vi "FRIC_navX_Internal_Serial_ProcessingLoop.vi"(7 "Device Number":T3, 11 "Rate (4Hz-200Hz)":u8=50 min=4 max=200) -> ()   [LabVIEW 2025]
doc: "This navX VI handles the reading/writing for the navX. All of the good stuff is in here.\nTHIS VI SHOULD NOT BE CALLED BY THE USER!"
uses:
  _TypeDefs/Z900_navX_SerialStreamTypeDef.ctl
  _TypeDefs/FRIC_navX_DeviceNumbersTypeDef.ctl
  <vilib>/Rock Robotics/WPI/SerialPort/WPI_SerialPort.ctl
  _TypeDefs/Z900_navX_ProtocolTypeDef.ctl
  _TypeDefs/FRIC_navX_ProcessingLoopStatesTypeDef_I2C.ctl
  _TypeDefs/FRIC_navX_I2C Process Loop TypeDef.ctl
  _TypeDefs/Z900_navX_DeviceTypeDef.ctl
  _TypeDefs/Z900_navX_NotifyPacketTypeDef.ctl
  _TypeDefs/Z900_navX_ActionTypeDef.ctl
  <vilib>/Rock Robotics/SystemInterfaces/i2clib/i2c_bus.ctl
  _TypeDefs/Z900_navX_IntegrationControlRegisters.ctl
  <vilib>/Rock Robotics/WPI/SPI/WPI_SPIDevRef.ctl
  <vilib>/Rock Robotics/SystemInterfaces/spilib/spi_bus.ctl
  <vilib>/Rock Robotics/WPI/SerialPort/WPI_SerialPortRef.ctl
  <vilib>/Platform/TimedLoop/XDataNode/timing_clust.ctl
  <vilib>/Platform/TimedLoop/XDataNode/nitl_modes.ctl
  <vilib>/Platform/TimedLoop/XDataNode/wakeup.ctl
  <vilib>/Rock Robotics/SystemInterfaces/NetworkCommunication/NetComm_UsageReport_ResourceType.ctl
  <vilib>/Rock Robotics/SystemInterfaces/Utilities/FPGA_UtilitiesRead LocalTime.vi
  <vilib>/Platform/TimedLoop/XDataNode/XDataNode.xnode
  <vilib>/Platform/TimedLoop/XDataNode/XDNodeRunTimeDep.lvlib
panel:
  in  "Tab Control":enum32{"Page 1", "Page 2"}(tab)
  in  "Halt":bool
  out "Connected":bool
  out "error":errorcluster
  in  "Stream Type":T1=enum."AHRSAndPositioning"
  in  "Serial Port":T2=enum."MXP TTL"
  out "Loop Time":i64
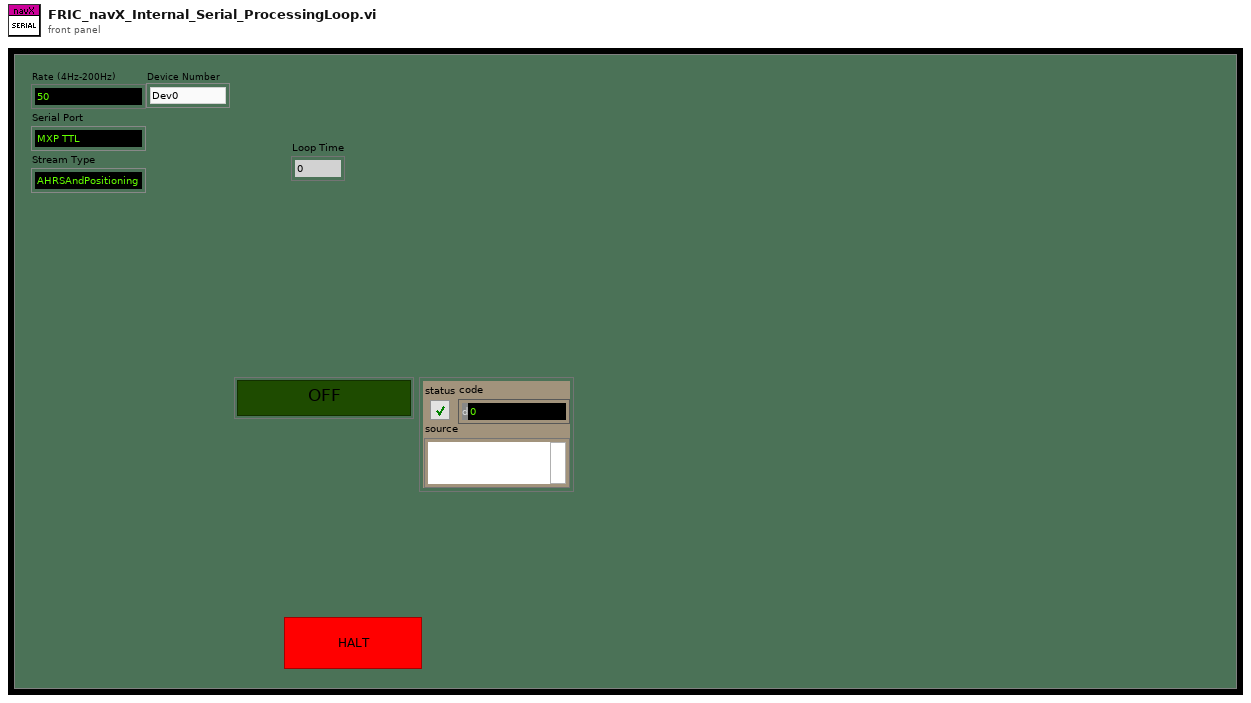
[diagram p1: front panel]
types:
  T1 = typedef "Z900_navX_SerialStreamTypeDef.ctl" = enum16{"YRPH", "Quaterinons", "Gyro/Raw", "AHRS", "AHRSAndPositioning", "AHRSAndPOSTime"}
  T2 = typedef "WPI_SerialPort.ctl" = enum16{"Onboard RS-232", "MXP TTL", "USB 1", "USB 2"}
  T3 = typedef "FRIC_navX_DeviceNumbersTypeDef.ctl" = enum16{"Dev0", "Dev1", "Dev2", "Dev3"}
  T4 = typedef "FRIC_navX_I2C Process Loop TypeDef.ctl" = cluster{"State Array":T5[], "error":errorcluster, "FPGA Cluster":cluster{"Last Valid FPGA Time":dbl, "Error Count":i32, "Initialized":bool}, "Device Info":T6, "I2CDevRef":cluster{"DevStatus":errorcluster, "Device Address":u8, "Handle":i32, "I2C Bus":T8}, "Registry":u8[], "Command Array":T9[], "Connected?":bool, "navX Device Memory Size":i32, "notification":T10, "Memory Size Set":bool, "SPIDevRef":T12, "navX Serial Open":cluster{"Stream Type":T1, "Serial Port":T2}, "SerialPortRef":T14, "Serial Read Buffer":string, "Serial Write Buffer":string[], "Device Number":T3, "navX SPI Open":cluster{"SPI Bus":T13, "Clock Rate (Hz)":dbl}, "Loop dt":i64, "current time":timestamp, "Loop Time":i64}
  T5 = typedef "FRIC_navX_ProcessingLoopStatesTypeDef_I2C.ctl" = enum16{"Process", "INI", "Check Packets Valid", "Close", "Clear VISA", "Generate Command", "Last Packet Valid", "Open", "Read", "Reset Serial", "Set Termination Char", "Update AE", "Wait", "Write", "Exit"}
  T6 = typedef "Z900_navX_DeviceTypeDef.ctl" = cluster{"Interface":cluster{"Protocol":T7, "Update Rate (4Hz-200Hz)":u8, "navX Open TypeDef":variant}, "Notify Packet":refnum<notifier>, "Loop VI Refnum":refnum<vi>, "Ready to Close Occurrence Refnum":refnum<k4>, "Name":string}
  T7 = typedef "Z900_navX_ProtocolTypeDef.ctl" = enum16{"SERIAL", "I2C", "SPI"}
  T8 = typedef "i2c_bus.ctl" = enum16{"I2C On-Board", "I2C MXP", "Invalid"}
  T9 = typedef "Z900_navX_IntegrationControlRegisters.ctl" = u8
  T10 = typedef "Z900_navX_NotifyPacketTypeDef.ctl" = cluster{"navX Action":T11, "Data":variant, "Stream Type":T1, "Device Number":T3}
  T11 = typedef "Z900_navX_ActionTypeDef.ctl" = enum16{"None", "Halt", "Normal Read", "Update Serial Protocol", "Update Rate Htz", "Zero-Yaw", "Zero-Displacement", "Zero-Velocity"}
  T12 = typedef "WPI_SPIDevRef.ctl" = cluster{"DevStatus":errorcluster, "Handle":i32, "SPI Bus":T13}
  T13 = typedef "spi_bus.ctl" = enum16{"SPI On-Board, CS0", "SPI On-Board, CS1", "SPI On-Board, CS2", "SPI On-Board, CS3", "SPI MXP", "Invalid"}
  T14 = typedef "WPI_SerialPortRef.ctl" = cluster{"DevStatus":errorcluster, "Serial Port Name":refnum<visa-resource-name>}
  T15 = typedef "XDNodeRunTimeDep.lvlib/timing_clust.ctl" = cluster{"Expected End [f-1]":u64, "Actual End [f-1]":u64, "Finished Late? [f-1]":bool, "Expected End [i-1]":u64, "Actual End [i-1]":u64, "Finished Late? [i-1]":bool, "Expected Start [i]":u64, "Actual Start [i]":u64, "Expected Start [f]":u64, "Actual Start [f]":u64, "Source Name":string, "Structure Name":string, "Period":i64, "Deadline":i64, "Offset":i64, "Start":i64, "Priority":i32, "Timeout":i32, "Mode":T16, "Wakeup Reason":T17, "Error":errorcluster, "Source Type":string, "Secondary Source Type":string, "Global End Time":u64, "Global Start Time":u64, "Frame Duration":u64, "Iteration Duration":u64, "Assigned CPU":i32, "I/O Scan Engine Mode":u32}
  T16 = typedef "XDNodeRunTimeDep.lvlib/nitl_modes.ctl" = enum32{"No Change", "Process missed periods, maintain original phase", "Discard missed periods, maintain original phase", "Process missed periods, ignore original phase", "Discard missed periods, ignore original phase"}
  T17 = typedef "XDNodeRunTimeDep.lvlib/wakeup.ctl" = enum32{"Normal", "Aborted", "Asynchronous wakeup", "Timing source error", "Timed loop error", "Timeout"}
  T18 = typedef "NetComm_UsageReport_ResourceType.ctl" = enum8{"Controller", "Module", "Language", "CANPlugin", "Accelerometer", "ADXL345", "AnalogChannel", "AnalogTrigger", "AnalogTriggerOutput", "CANJaguar", "Compressor", "Counter", "Dashboard", "DigitalInput", "DigitalOutput", "DriverStationCIO", "DriverStationEIO", "DriverStationLCD", "Encoder", "GearTooth", "Gyro", "I2C", "Framework", "Jaguar", "Joystick", "Kinect", "KinectStick", "PIDController", "Preferences", "PWM", "Relay", "RobotDrive", "SerialPort", "Servo", "Solenoid", "SPI", "Task", "Ultrasonic", "Victor", "Button", "Command", "AxisCamera", "PCVideoServer", "SmartDashboard", "Talon", "HiTechnicColorSensor", "HiTechnicAccel", "HiTechnicCompass", "SRF08", "AnalogOutput", "Victor SP", "Talon SRX", "CAN Talon SRX", "ADXL362 Accel", "ADXRS450 Gyro", "Rev SPARK", "Mindsensors SD540", "Digital Filter", "ADIS16448", "PDP", "PCM", "PigeonIMU", "Nidec Brushless", "CTRE CANifier", "CTRE TalonFX", "CTRE Future 1", "CTRE Future 2", "CTRE Future 3", "CTRE Future 4", "CTRE Future 5", "CTRE Future 6", "Linear Filter", "Xbox Controller", "USB Camera", "NavX", "Pixy", "Pixy2", "ScanseSweep", "Shuffleboard", "CAN", "Digilent DMC60", "PWM Victor SPX", "Rev SPARK MAX PWM", "Rev SPARK MAX CAN", "ADIS16470", "PIDController2", "ProfiledPIDController", "Kinematics", "Odometry", "Units", "Trapezoid Profile", "DutyCycle", "Addressable LEDs", "Fusion Venom", "CTRE Future 7", "CTRE Future 8", "CTRE Future 9", "CTRE Future 10", "CTRE Future 11", "CTRE Future 12", "CTRE Future 13", "CTRE Future 14", "Exponential Profile", "PS4 Controller", "Photon Camera", "Photon Pose Estimator", "Path Planner Path", "Path Planner Auto", "Path Finding Command", "Redux Future 1", "Redux Future 2", "Redux Future 3", "Redux Future 4", "Redux Future 5", "Rev SPARK Flex CAN", "Rev SPARK Flex PWM", "LEDPattern", "LinearQuadraticRegulator", "KalmanFilter", "PoseEstimator", "PoseEstimator3d", "LinearSystemLoop", "WPILib_future7", "WPILib_future8", "Rev_ServoHub", "YAMS", "LumenLabs_ConnectorX", "LumenLabs_ConnectorXLED"}
  T19 = cluster{"Last Valid FPGA Time":dbl, "Error Count":i32, "Initialized":bool}
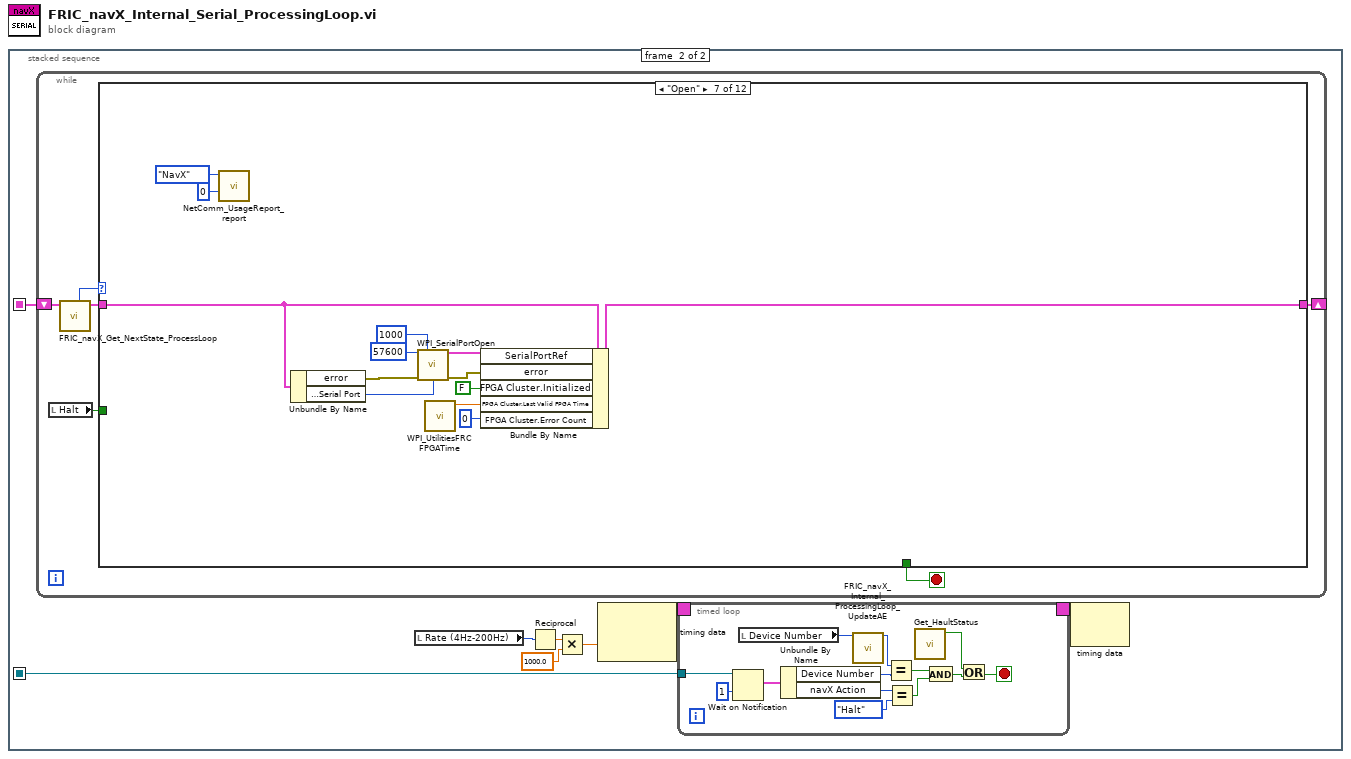
[diagram p0: block diagram]
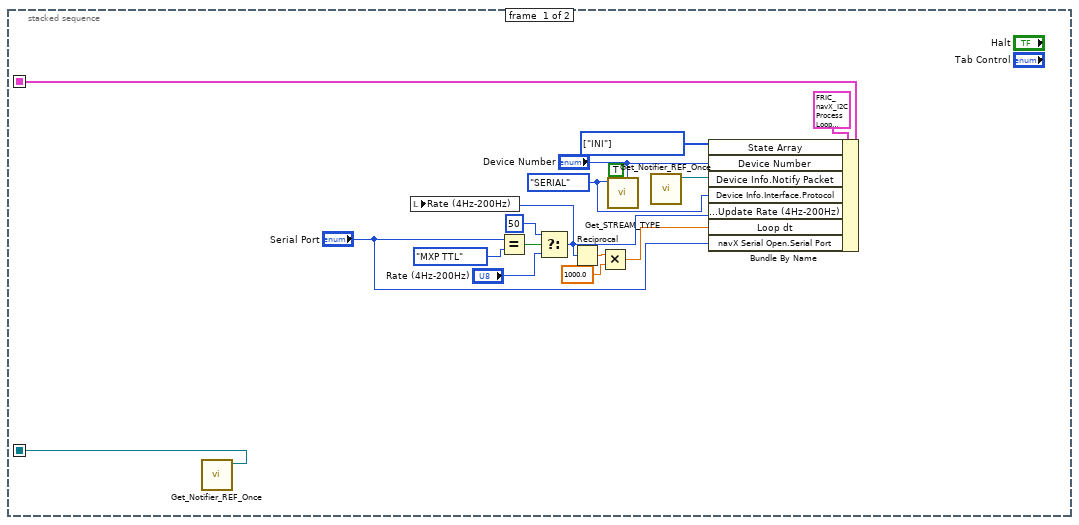
[diagram p2: hidden frame]
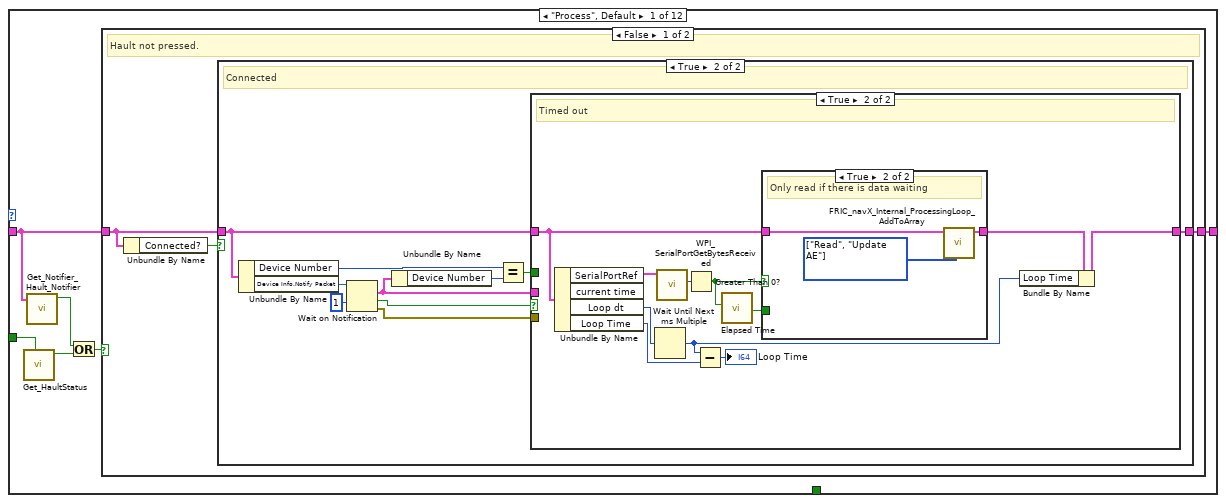
[diagram p3: hidden frame]
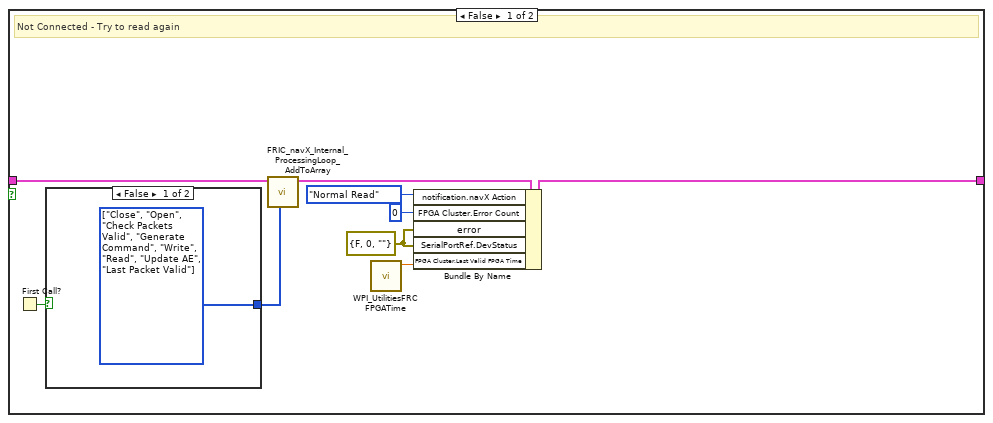
[diagram p4: hidden frame]
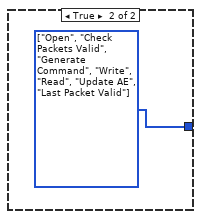
[diagram p5: hidden frame]
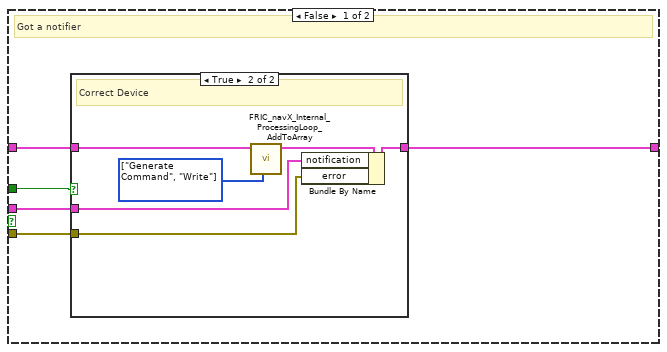
[diagram p6: hidden frame]
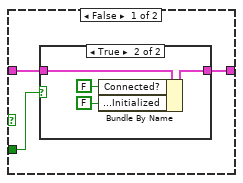
[diagram p8: hidden frame]
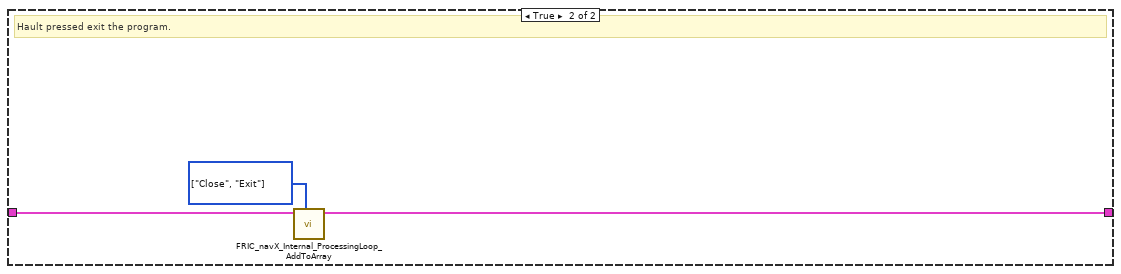
[diagram p10: hidden frame]
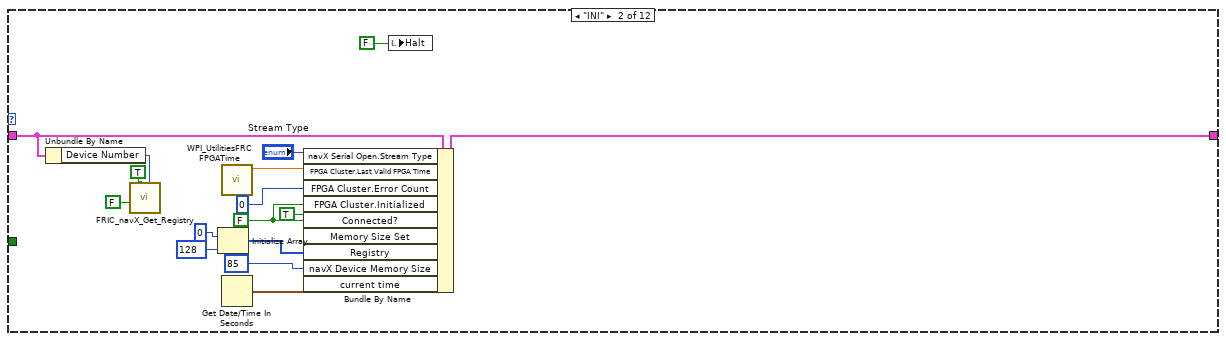
[diagram p11: hidden frame]
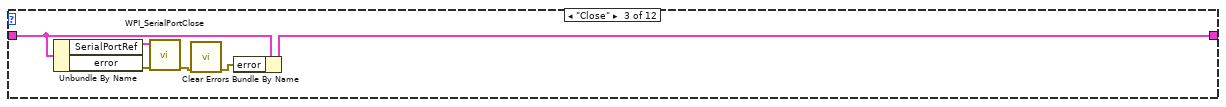
[diagram p12: hidden frame]
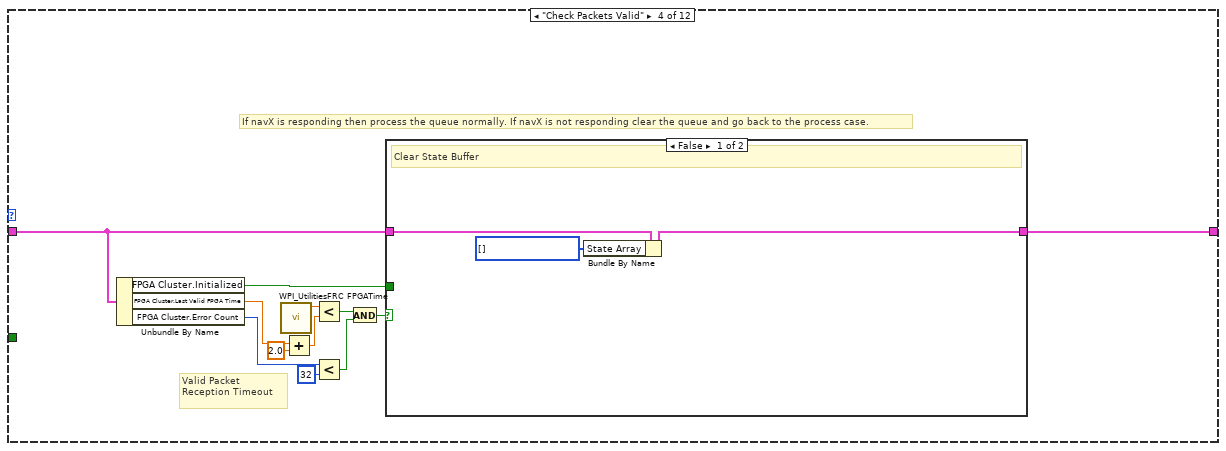
[diagram p13: hidden frame]
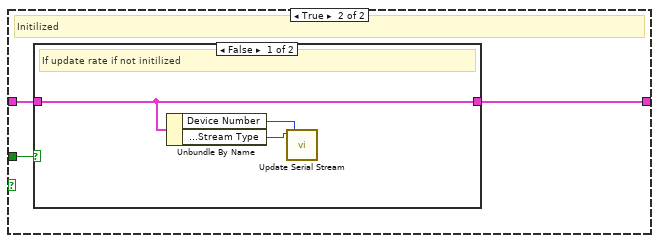
[diagram p14: hidden frame]
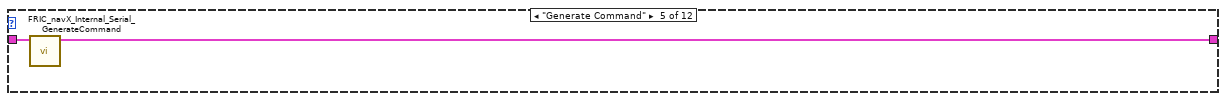
[diagram p16: hidden frame]
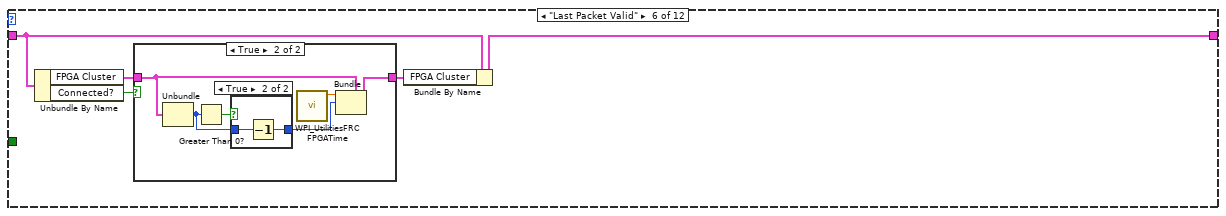
[diagram p17: hidden frame]
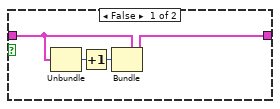
[diagram p18: hidden frame]
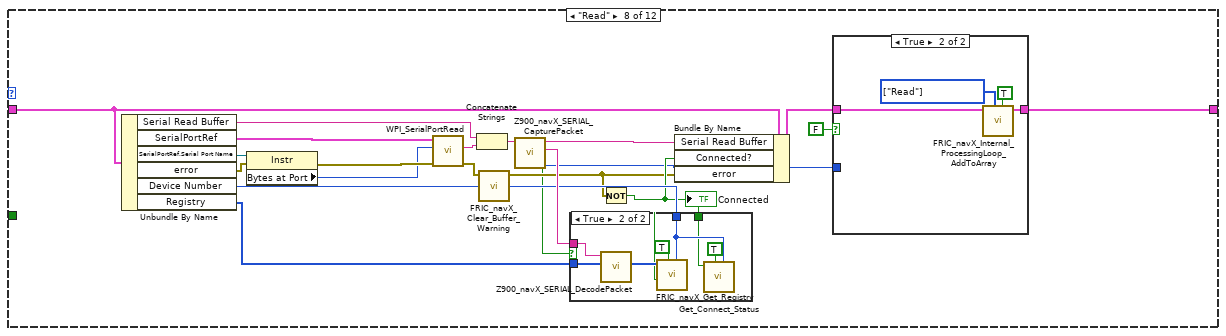
[diagram p20: hidden frame]
diagram:
  n1 = stacked-sequence {
    seq-local: [w17 _] -> [_ w25]
    seq-local: [w13 _] -> [_ w18]
    frame #0 {
      w1 = Z900_navX_ProtocolTypeDef."SERIAL" ("Protocol")
      w15 = T5[] [enum."INI"] items=["Process", "INI", "Check Packets Valid", "Close", "Clear VISA", "Generate Command", "Last Packet Valid", "Open", "Read", "Reset Serial", "Set Termination Char", "Update AE", "Wait", "Write", "Exit"] ("State Array")
      n2 = call "Get_Notifier_REF_Once.vi"() -> ("notifier ref out"=w13:refnum<notifier>)  [unwired: 10 in, 1 out]
      n3 = Equal?(x="Serial Port", y=WPI_SerialPort."MXP TTL") -> (x = y?=w11:bool)
      n4 = Select(t=u8 50, s=w11, f="Rate (4Hz-200Hz)") -> (s? t:f=w6:u8)
      n5 = local write "Rate (4Hz-200Hz)"(w6) -> ()
      n6 = Reciprocal(x=w6) -> (1/x=w9:dbl)
      n7 = Multiply(x=w9, y=1000.0) -> (x*y=w7:dbl)
      n8 = call "Get_STREAM_TYPE.vi"("Device Number"="Device Number", "Update"=TRUE, "Protocol (in)"=w1) -> ()  [unwired: 8 in, 1 out]
      n9 = call "Get_Notifier_REF_Once.vi"() -> ("notifier ref out"=w14:refnum<notifier>)  [unwired: 10 in, 1 out]
      n10 = Bundle By Name(cluster=T4 {"State Array"=[enum."INI", enum."Open"], "error"={"status"=FALSE, "code"=0, "source"=""}, "FPGA Cluster"={"Last Valid FPGA Time"=0.0, "Error Count"=0, "Initialized"=FALSE}, "Device Info"={"Interface"={"Protocol"=enum."SERIAL", "Update Rate (4Hz-200Hz)"=4, "navX Open TypeDef"=variant}, "Notify Packet"=refnum, "Loop VI Refnum"=refnum, "Ready to Close Occurrence Refnum"=refnum, "Name"=""}, "I2CDevRef"={"DevStatus"={"status"=FALSE, "code"=0, "source"=""}, "Device Address"=0, "Handle"=0, "I2C Bus"=enum."Invalid"}, "Registry"=[], "Command Array"=[214, 32], "Connected?"=FALSE, "navX Device Memory Size"=85, "notification"={"navX Action"=enum."None", "Data"=variant, "Stream Type"=enum."YRPH", "Device Number"=enum."Dev0"}, "Memory Size Set"=FALSE, "SPIDevRef"={"DevStatus"={"status"=FALSE, "code"=0, "source"=""}, "Handle"=0, "SPI Bus"=enum."SPI On-Board, CS0"}, "navX Serial Open"={"Stream Type"=enum."YRPH", "Serial Port"=enum."Onboard RS-232"}, "SerialPortRef"={"DevStatus"={"status"=FALSE, "code"=0, "source"=""}, "Serial Port Name"=""}, "Serial Read Buffer"="", "Serial Write Buffer"=[], "Device Number"=enum."Dev0", "navX SPI Open"={"SPI Bus"=enum."SPI MXP", "Clock Rate (Hz)"=500000.0}, "Loop dt"=0, "current time"=timestamp(0 s since 1904-01-01), "Loop Time"=0} ("I2C Process Loop TypeDef"), "State Array"=w15, "Device Number"="Device Number", "Device Info.Notify Packet"=w14, "Device Info.Interface.Protocol"=w1, "Device Info.Interface.Update Rate (4Hz-200Hz)"=w6, "Loop dt"=w7, "navX Serial Open.Serial Port"="Serial Port") -> (w17:T4)
    }
    frame #1 {
      n11 = while {
        shift-right: [w45] -> _
        shift-left: w25 -> [w48]
        stop <- w49 stop-if-true
        n12 = local read "Halt"() -> (w44:bool)
        n13 = call "FRIC_navX_Get_NextState_ProcessLoop.vi"("I2C Process Loop TypeDef (in)"=w48) -> ("I2C Process Loop TypeDef (out)"=w47:T4, "Current State"=w46:T5)  [unwired: 9 in]
        n14 = case shown="\"Open\"" w46 {
          tunnel: [_ _ _ _ _ _ _ _ _ _ TRUE _] -> w49
          tunnel: w47 -> [w53 w121 w138 w142 w162 w166 w193 w204 w231 w244 w251 w259]
          tunnel: [w55 w128 w137 w143 w161 w165 w192 w202 w232 w233 w251 w259] -> w45
          tunnel: w44 -> [w54 _ _ _ _ _ _ _ _ _ _ _]
          frame "Process", Default {
            n15 = call "Get_HaultStatus.vi"("Update"=w54) -> ("Hault"=w51:bool)  [unwired: 10 in]
            n16 = call "Get_Notifier_Hault_Notifier.vi"("Process Loop TypeDef (in)"=w53) -> ("Hault Notifier"=w52:bool)  [unwired: 10 in]
            n17 = Or(x=w52, y=w51) -> (x .or. y?=w50:bool)
            n18 = case shown="False" w50 {
              tunnel: [w58 w115] -> w55
              tunnel: w53 -> [w56 w116]
              frame False {
                # "Hault not pressed."
                n19 = Unbundle By Name(w56) -> ("Connected?"=w57:bool)
                n20 = case shown="True" w57 {
                  tunnel: w56 -> [w67 w78]
                  tunnel: [w64 w79] -> w58
                  frame False {
                    w60 = errorcluster {"status"=FALSE, "code"=0, "source"=""} ("error")
                    # "Not Connected - Try to read again"
                    n21 = First Call?() -> (First Call?: T/F=w61:bool)
                    n22 = case shown="False" w61 {
                      tunnel: [w68 w69] -> w66
                      frame False {
                        w68 = T5[] [enum."Close", enum."Open", enum."Check Packets Valid", enum."Generate Command", enum."Write", enum."Read", enum."Update AE", enum."Last Packet Valid"] items=["Process", "INI", "Check Packets Valid", "Close", "Clear VISA", "Generate Command", "Last Packet Valid", "Open", "Read", "Reset Serial", "Set Termination Char", "Update AE", "Wait", "Write", "Exit"]
                      }
                      frame True {
                        w69 = T5[] [enum."Open", enum."Check Packets Valid", enum."Generate Command", enum."Write", enum."Read", enum."Update AE", enum."Last Packet Valid"] items=["Process", "INI", "Check Packets Valid", "Close", "Clear VISA", "Generate Command", "Last Packet Valid", "Open", "Read", "Reset Serial", "Set Termination Char", "Update AE", "Wait", "Write", "Exit"]
                      }
                    }
                    n23 = call "FRIC_navX_Internal_ProcessingLoop_AddToArray.vi"("States Array"=w66, "I2C Process Loop TypeDef (in)"=w67) -> ("I2C Process Loop TypeDef (out)"=w65:T4)  [unwired: 9 in]
                    n24 = call <vilib>:"WPI_UtilitiesFRC FPGATime.vi"() -> ("FPGA Time"=w59:dbl)  [unwired: 10 in, 1 out]
                    n25 = Bundle By Name(cluster=w65, "notification.navX Action"=Z900_navX_ActionTypeDef."Normal Read", "FPGA Cluster.Error Count"=0, "error"=w60, "SerialPortRef.DevStatus"=w60, "FPGA Cluster.Last Valid FPGA Time"=w59) -> (w64:T4)
                  }
                  frame True {
                    # "Connected"
                    n26 = Unbundle By Name(w78) -> ("Device Number"=w72:T3, "Device Info.Notify Packet"=w77:refnum<notifier>)
                    n27 = Wait on Notification(notifier=w77, timeout in ms (-1)=1) -> (notification=w73:T10, timed out?=w74:bool, error out=w75:errorcluster)  [unwired: 2 in, 1 out]
                    n28 = Unbundle By Name(w73) -> ("Device Number"=w71:T3)
                    n29 = Equal?(x=w72, y=w71) -> (x = y?=w70:bool)
                    n30 = case shown="True" w74 {
                      tunnel: w78 -> [w84 w99]
                      tunnel: [w83 w96] -> w79
                      tunnel: w73 -> [w82 _]
                      tunnel: w75 -> [w81 _]
                      tunnel: w70 -> [w80 _]
                      frame False {
                        # "Got a notifier"
                        n31 = case shown="True" w80 {
                          tunnel: w84 -> [w85 w91]
                          tunnel: [w85 w90] -> w83
                          tunnel: w82 -> [_ w89]
                          tunnel: w81 -> [_ w86]
                          frame False {
                          }
                          frame True {
                            w87 = T5[] [enum."Generate Command", enum."Write"] items=["Process", "INI", "Check Packets Valid", "Close", "Clear VISA", "Generate Command", "Last Packet Valid", "Open", "Read", "Reset Serial", "Set Termination Char", "Update AE", "Wait", "Write", "Exit"] ("States Array")
                            # "Correct Device"
                            n32 = call "FRIC_navX_Internal_ProcessingLoop_AddToArray.vi"("States Array"=w87, "I2C Process Loop TypeDef (in)"=w91) -> ("I2C Process Loop TypeDef (out)"=w88:T4)  [unwired: 9 in]
                            n33 = Bundle By Name(cluster=w88, "notification"=w89, "error"=w86) -> (w90:T4)
                          }
                        }
                      }
                      frame True {
                        # "Timed out"
                        n34 = Unbundle By Name(w99) -> ("SerialPortRef"=w101:T14, "Loop dt"=w95:i64, "Loop Time"=w93:i64)  [unwired: 1 out]
                        n35 = Wait Until Next ms Multiple(millisecond multiple=w95) -> (millisecond timer value=w94:u32)
                        n36 = call <vilib>:"WPI_SerialPortGetBytesReceived.vi"("SerialPortRef"=w101) -> ("Bytes at Port"=w100:u32)  [unwired: 8 in, 2 out]
                        n37 = Greater Than 0?(x=w100) -> (x > 0?=w98:bool)
                        n38 = Subtract(x=w94, y=w93) -> (x-y=→"Loop Time":i64)
                        n39 = call "Elapsed Time"("Reset"=w98) -> ("Time has Elapsed"=w97:bool)  [unwired: 11 in, 7 out]
                        n40 = case shown="True" w98 {
                          tunnel: [w103 w112] -> w102
                          tunnel: w99 -> [w104 w111]
                          tunnel: w97 -> [w105 _]
                          frame False {
                            n41 = case shown="True" w105 {
                              tunnel: w104 -> [w106 w110]
                              tunnel: [w106 w109] -> w103
                              frame False {
                              }
                              frame True {
                                n42 = Bundle By Name(cluster=w110, "Connected?"=FALSE, "FPGA Cluster.Initialized"=FALSE) -> (w109:T4)
                              }
                            }
                          }
                          frame True {
                            w113 = T5[] [enum."Read", enum."Update AE"] items=["Process", "INI", "Check Packets Valid", "Close", "Clear VISA", "Generate Command", "Last Packet Valid", "Open", "Read", "Reset Serial", "Set Termination Char", "Update AE", "Wait", "Write", "Exit"]
                            # "Only read if there is data waiting"
                            n43 = call "FRIC_navX_Internal_ProcessingLoop_AddToArray.vi"("States Array"=w113, "I2C Process Loop TypeDef (in)"=w111) -> ("I2C Process Loop TypeDef (out)"=w112:T4)  [unwired: 9 in]
                          }
                        }
                        n44 = Bundle By Name(cluster=w102, "Loop Time"=w94) -> (w96:T4)
                      }
                    }
                  }
                }
              }
              frame True {
                w114 = T5[] [enum."Close", enum."Exit"] items=["Process", "INI", "Check Packets Valid", "Close", "Clear VISA", "Generate Command", "Last Packet Valid", "Open", "Read", "Reset Serial", "Set Termination Char", "Update AE", "Wait", "Write", "Exit"] ("States Array")
                # "Hault pressed exit the program."
                n45 = call "FRIC_navX_Internal_ProcessingLoop_AddToArray.vi"("States Array"=w114, "I2C Process Loop TypeDef (in)"=w116) -> ("I2C Process Loop TypeDef (out)"=w115:T4)  [unwired: 9 in]
              }
            }
          }
          frame "INI" {
            w126 = FALSE ("Initialized")
            n46 = Unbundle By Name(w121) -> ("Device Number"=w120:T3)
            n47 = call "FRIC_navX_Get_Registry.vi"("Device Number"=w120, "Update"=TRUE, "Connected?"=FALSE) -> ()  [unwired: 7 in, 2 out]
            n48 = Initialize Array(u8 0 ("Received Data"), 128 ("hex")) -> (w124:u8[])
            n49 = call <vilib>:"WPI_UtilitiesFRC FPGATime.vi"() -> ("FPGA Time"=w130:dbl)  [unwired: 10 in, 1 out]
            n50 = Get Date/Time In Seconds() -> (seconds since 1Jan1904=w117:timestamp)
            n51 = Bundle By Name(cluster=w121, "navX Serial Open.Stream Type"="Stream Type", "FPGA Cluster.Last Valid FPGA Time"=w130, "FPGA Cluster.Error Count"=0 ("Error Count"), "FPGA Cluster.Initialized"=w126, "Connected?"=w126, "Memory Size Set"=TRUE, "Registry"=w124, "navX Device Memory Size"=85 ("hex"), "current time"=w117) -> (w128:T4)
            n52 = local write "Halt"(FALSE ("Halt")) -> ()
          }
          frame "Close" {
            n53 = Unbundle By Name(w138) -> ("SerialPortRef"=w135:T14, "error"=w134:errorcluster)
            n54 = call <vilib>:"WPI_SerialPortClose.vi"("error in (no error)"=w134, "SerialPortRef"=w135) -> ("error out"=w133:errorcluster)  [unwired: 9 in]
            n55 = call <vilib>:"Clear Errors.vi"("error in (no error)"=w133) -> ("error out"=w136:errorcluster)  [unwired: 5 in, 1 out]
            n56 = Bundle By Name(cluster=w138, "error"=w136) -> (w137:T4)
          }
          frame "Check Packets Valid" {
            # "If navX is responding then process the queue normally. If navX is not responding clear the queue and go back to the process case."
            # "Valid Packet Reception Timeout"
            n57 = Unbundle By Name(w142) -> ("FPGA Cluster.Initialized"=w140:bool, "FPGA Cluster.Last Valid FPGA Time"=w141:dbl, "FPGA Cluster.Error Count"=w139:i32)
            n58 = call <vilib>:"WPI_UtilitiesFRC FPGATime.vi"() -> ("FPGA Time"=w148:dbl)  [unwired: 10 in, 1 out]
            n59 = Add(x=w141, y=2.0) -> (x+y=w149:dbl)
            n60 = Less?(x=w148, y=w149) -> (x < y?=w146:bool)
            n61 = Less?(x=w139, y=32) -> (x < y?=w145:bool)
            n62 = And(x=w146, y=w145) -> (x .and. y?=w144:bool)
            n63 = case shown="False" w144 {
              tunnel: w142 -> [w153 w156]
              tunnel: [w152 w155] -> w143
              tunnel: w140 -> [_ w154]
              frame False {
                w151 = T5[] [] items=["Process", "INI", "Check Packets Valid", "Close", "Clear VISA", "Generate Command", "Last Packet Valid", "Open", "Read", "Reset Serial", "Set Termination Char", "Update AE", "Wait", "Write", "Exit"] ("f")
                # "Clear State Buffer"
                n64 = Bundle By Name(cluster=w153, "State Array"=w151) -> (w152:T4)
              }
              frame True {
                # "Initilized"
                n65 = case shown="False" w154 {
                  tunnel: w156 -> [w159 w160]
                  tunnel: [w159 w160] -> w155
                  frame False {
                    # "If update rate if not initilized"
                    n66 = Unbundle By Name(w159) -> ("Device Number"=w158:T3, "navX Serial Open.Stream Type"=w157:T1)
                    n67 = call "Update Serial Stream.vi"("Device Number"=w158, "Stream Type"=w157) -> ()  [unwired: 10 in]
                  }
                  frame True {
                    # "Everything is good keep going"
                  }
                }
              }
            }
          }
          frame "Generate Command" {
            n68 = call "FRIC_navX_Internal_Serial_GenerateCommand.vi"("Serial Process Loop TypeDef (in)"=w162) -> ("Serial Process Loop TypeDef (out)"=w161:T4)  [unwired: 10 in]
          }
          frame "Last Packet Valid" {
            n69 = Unbundle By Name(w166) -> ("FPGA Cluster"=w167:T19, "Connected?"=w163:bool)
            n70 = case shown="True" w163 {
              tunnel: [w170 w177] -> w164
              tunnel: w167 -> [w169 w173]
              frame False {
                n71 = Unbundle(w169) -> ("Error Count"=w168:i32)  [unwired: 2 out]
                n72 = Increment(x=w168) -> (x+1=w171:i32)
                n73 = Bundle(cluster=w169, "Error Count"=w171) -> (w170:T19)  [unwired: 2 in]
              }
              frame True {
                n74 = Unbundle(w173) -> ("Error Count"=w172:i32)  [unwired: 2 out]
                n75 = Greater Than 0?(x=w172) -> (x > 0?=w175:bool)
                n76 = case shown="True" w175 {
                  tunnel: [w178 w180] -> w174
                  tunnel: w172 -> [w178 w179]
                  frame False {
                  }
                  frame True {
                    n77 = Decrement(x=w179) -> (x-1=w180:i32)
                  }
                }
                n78 = call <vilib>:"WPI_UtilitiesFRC FPGATime.vi"() -> ("FPGA Time"=w176:dbl)  [unwired: 10 in, 1 out]
                n79 = Bundle(cluster=w173, "Last Valid FPGA Time"=w176, "Error Count"=w174) -> (w177:T19)  [unwired: 1 in]
              }
            }
            n80 = Bundle By Name(cluster=w166, "FPGA Cluster"=w164) -> (w165:T4)
          }
          frame "Open" {
            n81 = call <vilib>:"NetComm_UsageReport_report.vi"("Instance Number"=u8 0, "Resource Type"=NetComm_UsageReport_ResourceType."NavX") -> ()  [unwired: 10 in]
            n82 = Unbundle By Name(w193) -> ("error"=w184:errorcluster, "navX Serial Open.Serial Port"=w183:T2)
            n83 = call <vilib>:"WPI_SerialPortOpen.vi"("Baud Rate"=u32 57600, "Timeout Value (ms)"=u32 1000, "error in (no error)"=w184, "Serial Port"=w183) -> ("SerialPortRef"=w187:T14, "error out"=w188:errorcluster)  [unwired: 10 in]
            n84 = call <vilib>:"WPI_UtilitiesFRC FPGATime.vi"() -> ("FPGA Time"=w186:dbl)  [unwired: 10 in, 1 out]
            n85 = Bundle By Name(cluster=w193, "SerialPortRef"=w187, "error"=w188, "FPGA Cluster.Initialized"=FALSE ("Initialized"), "FPGA Cluster.Last Valid FPGA Time"=w186, "FPGA Cluster.Error Count"=0) -> (w192:T4)
          }
          frame "Read" {
            n86 = Unbundle By Name(w204) -> ("Serial Read Buffer"=w210:string, "SerialPortRef"=w211:T14, "SerialPortRef.Serial Port Name"=w214:refnum<visa-resource-name>, "error"=w213:errorcluster, "Device Number"=w201:T3, "Registry"=w206:u8[])
            n87 = property class="Instr"(reference=w214, error in=w213) -> (error out=w208:errorcluster, "Bytes at Port"=w195:u32)  [unwired: 1 in]
            n88 = call <vilib>:"WPI_SerialPortRead.vi"("error in (no error)"=w208, "Num Bytes to Read"=w195, "SerialPortRef"=w211) -> ("error out"=w198:errorcluster, "Buffer"=w212:string)  [unwired: 6 in, 1 out]
            n89 = Concatenate Strings(w210, w212) -> (w209:string)
            n90 = call "FRIC_navX_Clear_Buffer_Warning.vi"("error in"=w198) -> ("error out"=w197:errorcluster)  [unwired: 10 in]
            n91 = call "Z900_navX_SERIAL_CapturePacket.vi"("Buffer"=w209) -> ("Packet Size"=w199:i32, "Packet Located"=w196:bool, "Packet"=w205:string, "Buffer"=w207:string)  [unwired: 7 in]
            n92 = Not(x=w197) -> (.not. x?=w200:bool)
            "Connected" <- w200
            n93 = case shown="True" w196 {
              tunnel: w206 -> [_ w220]
              tunnel: w205 -> [_ w219]
              tunnel: w201 -> [_ w217]
              tunnel: w200 -> [_ w216]
              frame False {
              }
              frame True {
                n94 = call "Z900_navX_SERIAL_DecodePacket.vi"("Data (in)"=w220, "Packet (in)"=w219) -> ("Data"=w221:u8[])  [unwired: 7 in, 2 out]
                n95 = call "FRIC_navX_Get_Registry.vi"("Device Number"=w217, "Update"=TRUE, "Connected?"=w216, "Registry (in)"=w221) -> ()  [unwired: 6 in, 2 out]
                n96 = call "Get_Connect_Status.vi"("Device Number"=w217, "Update"=TRUE, "Connected"=w216) -> ()  [unwired: 8 in, 1 out]
              }
            }
            n97 = Bundle By Name(cluster=w204, "Serial Read Buffer"=w207, "Connected?"=w200, "error"=w197) -> (w203:T4)
            n98 = case shown="True" FALSE {
              tunnel: w203 -> [w222 w226]
              tunnel: [w222 w225] -> w202
              tunnel: w199 -> [_ _]
              frame False {
              }
              frame True {
                w224 = T5[] [enum."Read"] items=["Process", "INI", "Check Packets Valid", "Close", "Clear VISA", "Generate Command", "Last Packet Valid", "Open", "Read", "Reset Serial", "Set Termination Char", "Update AE", "Wait", "Write", "Exit"] ("States Array")
                n99 = call "FRIC_navX_Internal_ProcessingLoop_AddToArray.vi"("Add to beginning"=TRUE, "States Array"=w224, "I2C Process Loop TypeDef (in)"=w226) -> ("I2C Process Loop TypeDef (out)"=w225:T4)  [unwired: 8 in]
              }
            }
          }
          frame "Reset Serial" {
            n100 = Unbundle By Name(w231) -> ("SerialPortRef"=w230:T14, "error"=w228:errorcluster)
            n101 = call <vilib>:"WPI_SerialPortReset.vi"("error in (no error)"=w228, "SerialPortRef"=w230) -> ("error out"=w227:errorcluster, "SerialPortRef"=w229:T14)  [unwired: 8 in]
            n102 = Bundle By Name(cluster=w231, "SerialPortRef"=w229, "error"=w227) -> (w232:T4)
          }
          frame "Write" {
            n103 = Unbundle By Name(w244) -> ("SerialPortRef"=w242:T14, "Serial Write Buffer"=w239:string[], "SerialPortRef.DevStatus"=w243:errorcluster)
            n104 = Delete From Array(array=w239, index=0) -> (deleted portion=w238:string, array with subset deleted=w235:string[])  [unwired: 1 in]
            n105 = call <vilib>:"WPI_SerialPortWrite.vi"("error in (no error)"=w243, "Buffer"=w238, "SerialPortRef"=w242) -> ("error out"=w241:errorcluster, "SerialPortRef"=w240:T14)  [unwired: 6 in, 1 out]
            n106 = Empty Array?(array=w235) -> (empty?=w234:bool)
            n107 = Bundle By Name(cluster=w244, "SerialPortRef"=w240, "error"=w241, "Serial Write Buffer"=w235) -> (w236:T4)
            n108 = case shown="False" w234 {
              tunnel: [w248 w249] -> w233
              tunnel: w236 -> [w247 w249]
              frame False {
                w246 = T5[] [enum."Write"] items=["Process", "INI", "Check Packets Valid", "Close", "Clear VISA", "Generate Command", "Last Packet Valid", "Open", "Read", "Reset Serial", "Set Termination Char", "Update AE", "Wait", "Write", "Exit"] ("States Array")
                # "Write again because buffer is not empty."
                n109 = call "FRIC_navX_Internal_ProcessingLoop_AddToArray.vi"("Add to beginning"=TRUE, "States Array"=w246, "I2C Process Loop TypeDef (in)"=w247) -> ("I2C Process Loop TypeDef (out)"=w248:T4)  [unwired: 8 in]
              }
              frame True {
                # "Process the rest of the state array"
              }
            }
          }
          frame "Exit" {
            n110 = Unbundle By Name(w251) -> ("Device Info"=w250:T6)
            n111 = in-place {
              in-place-border: w250 -> [w254]
              # "Set Occurence of Close"
              n112 = Unbundle By Name(w254) -> ("Ready to Close Occurrence Refnum"=w255:refnum<k4>)
              n113 = local write "Halt"(FALSE ("Halt")) -> ()
              n114 = Set Occurrence(w255) -> ()
            }
          }
          frame "Update AE" {
            n115 = Unbundle By Name(w259) -> ("Device Number"=w257:T3, "error"=w258:errorcluster)
            "error" <- w258
            n116 = call "Get_Error_Status.vi"("Device Number"=w257, "Update"=TRUE, "error in"=w258) -> ()  [unwired: 8 in, 1 out]
          }
        }
      }
      n117 = local read "Rate (4Hz-200Hz)"() -> (w23:u8)
      n118 = Reciprocal(x=w23) -> (1/x=w22:dbl)
      n119 = Multiply(x=w22, y=1000.0) -> (x*y=w19:dbl)
      n120 = node-c288(w19) -> (w21:T15)  [unwired: 1 in]
      n121 = timed-loop {
        timing: w21 -> [_]
        timing-out: [_] -> w20
        tunnel: w18 -> [w29]
        stop <- w28 stop-if-true
        n122 = Wait on Notification(notifier=w29, timeout in ms (-1)=1) -> (notification=w34:T10)  [unwired: 2 in, 3 out]
        n123 = local read "Device Number"() -> (w32:T3)
        n124 = Unbundle By Name(w34) -> ("Device Number"=w33:T3, "navX Action"=w36:T11)
        n125 = call "FRIC_navX_Internal_ProcessingLoop_UpdateAE.vi"("Device Number"=w32) -> ()  [unwired: 15 in]
        n126 = Equal?(x=w32, y=w33) -> (x = y?=w31:bool)
        n127 = Equal?(x=w36, y=Z900_navX_ActionTypeDef."Halt") -> (x = y?=w30:bool)
        n128 = call "Get_HaultStatus.vi"() -> ("Hault"=w27:bool)  [unwired: 11 in]
        n129 = And(x=w31, y=w30) -> (x .and. y?=w26:bool)
        n130 = Or(x=w27, y=w26) -> (x .or. y?=w28:bool)
      }
      n131 = node-c288(w20) -> ()  [unwired: 1 out]
    }
  }
